vi "Interface _Envio_Recepcion.vi"() -> ()   [LabVIEW 2017]
uses:
  <vilib>/Instr/_visa.llb/VISA Configure Serial Port (Instr).vi
panel:
  out "Acelerómetro Carga 4":waveform(dbl)(graph)
  out "Acelerómetro Eje 2":waveform(dbl)(graph)
  out "Acelerómetro Eje 3":waveform(dbl)(graph)
  out "return count":u32
  in  "Delay":u32
  out "Acelerómetro Motor 1":waveform(dbl)(graph)
  in  "Resetear Gráficos":bool
  out "Datos Crudos":string
  in  "Paro de emergencia":bool
  out "Status":bool
  out "Tasa de muestreo (Hz)":dbl(knob) scale=0.0..1.0
  in  "Puerto COM":refnum<visa-resource-name>
  out "String":string
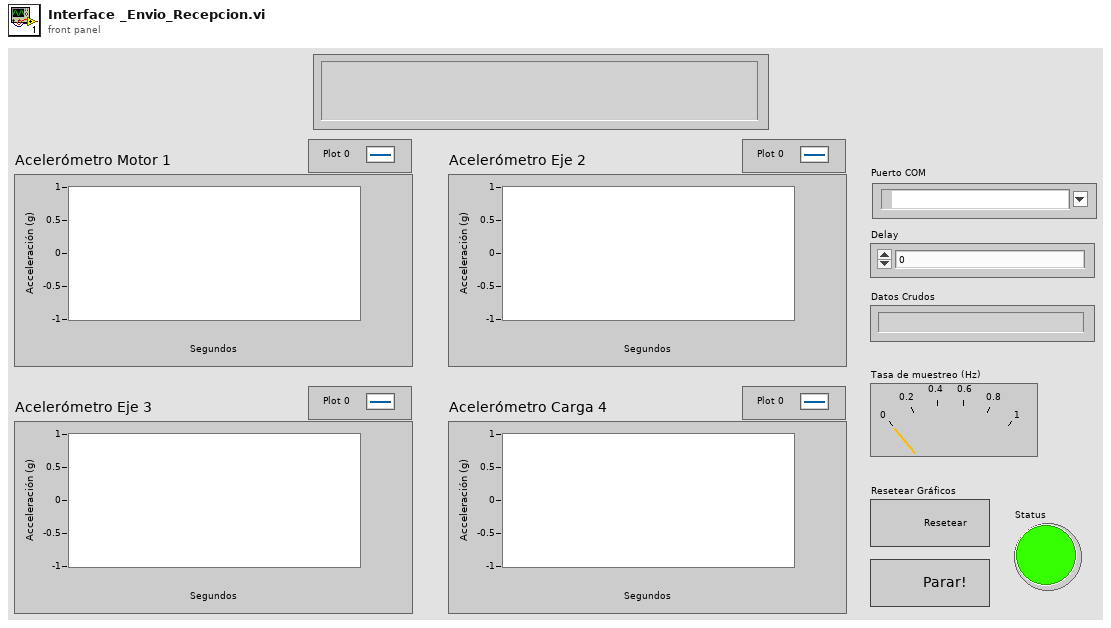
[diagram p1: front panel]
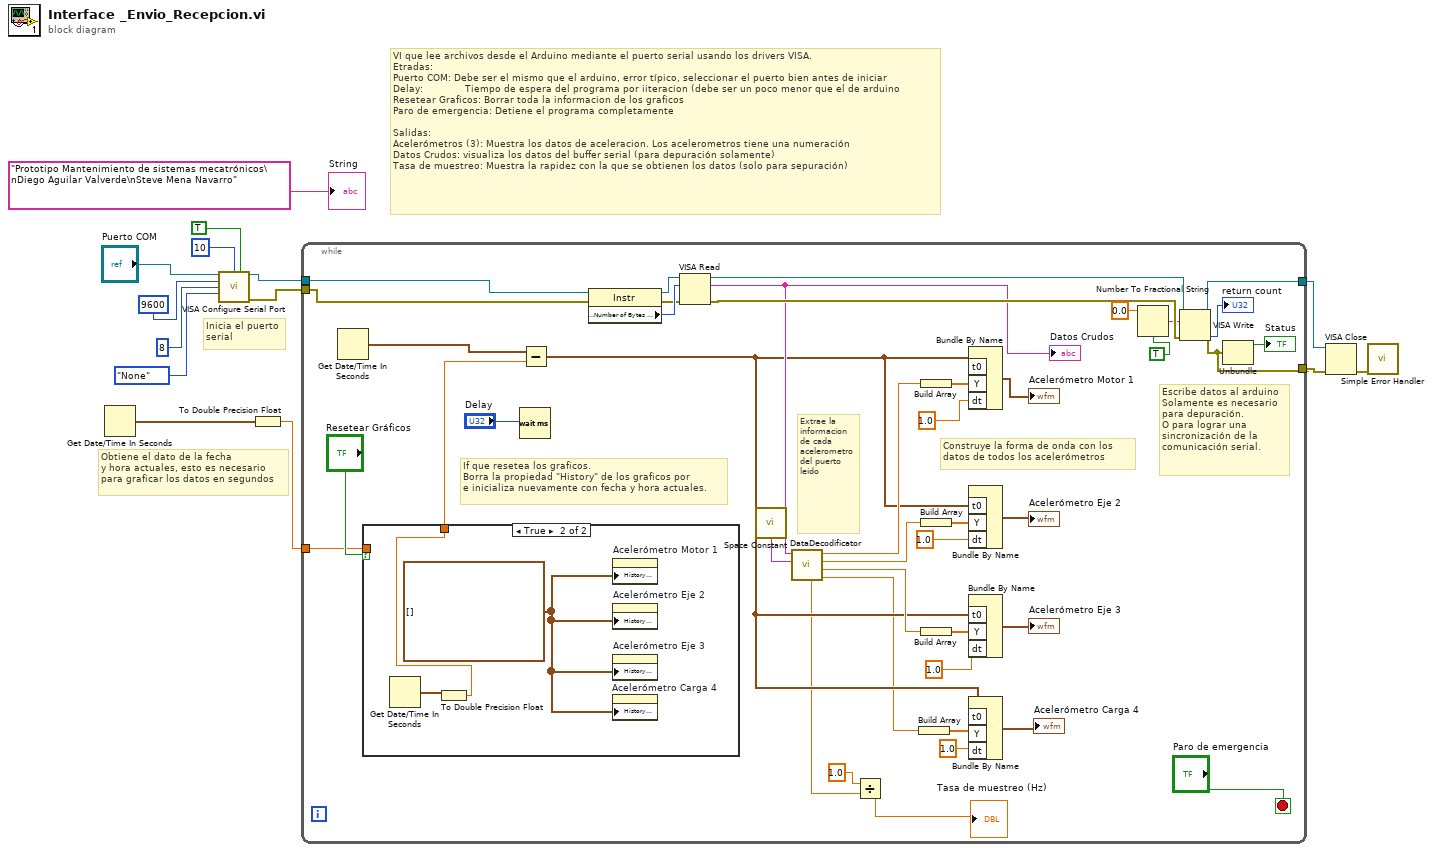
[diagram p0: block diagram]
diagram:
  # "Obtiene el dato de la fecha \ny hora actuales, esto es necesario\npara graficar los datos en segundos"
  # "Inicia el puerto\nserial"
  # "VI que lee archivos desde el Arduino mediante el puerto serial usando los drivers VISA.\nEtradas:\nPuerto COM: Debe ser el mismo que el arduino, error típico, seleccionar el puerto bien antes de iniciar\nDelay:              Tiempo de espera del programa por iiteracion (debe ser un poco menor que el de arduino\nResetear Graficos: Borrar toda la informacion de los graficos\nParo de emergencia: Detiene el programa completamente\n\nSalidas: \nAcelerómetros (3): Muestra los datos de aceleracion. Los acelerometros tiene una numeración\nDatos Crudos: visualiza los datos del buffer serial (para depuración solamente)\nTasa de muestreo: Muestra la rapidez con la que se obtienen los datos (solo para sepuración)"
  n1 = Get Date/Time In Seconds() -> (seconds since 1Jan1904=w1:timestamp)
  n2 = call-poly "VISA Configure Serial Port"("VISA resource name"="Puerto COM", "termination char\n(0xA = '\\n' = LF)"=u8 10 ("termination char\n(0xA = '\\n' = LF)"), "Enable Termination\nChar (T)"=TRUE ("Enable Termination\nChar (T)"), "baud rate (9600)"=u32 9600, "data bits (8)"=u16 8, "parity (0:none)"=enum16{"None", "Odd", "Even", "Mark", "Space"}."None") -> ("VISA resource name out"=w8:refnum<visa-resource-name>, "error out"=w7:errorcluster)  [unwired: 8 in]
  n3 = To Double Precision Float(number=w1) -> (double precision float=w2:dbl)
  n4 = while {
    tunnel: w8 -> [w56]
    tunnel: w7 -> [w55]
    tunnel: [w37] -> w6
    tunnel: [w35] -> w5
    tunnel: w2 -> [w40]
    stop <- "Paro de emergencia" stop-if-true
    # "Escribe datos al arduino\nSolamente es necesario \npara depuración. \nO para lograr una \nsincronización de la \ncomunicación serial."
    # "Extrae la informacion de cada acelerometro del puerto leído"
    # "Construye la forma de onda con los \ndatos de todos los acelerómetros"
    # "If que resetea los graficos.\nBorra la propiedad \"History\" de los graficos por\ne inicializa nuevamente con fecha y hora actuales."
    n5 = Get Date/Time In Seconds() -> (seconds since 1Jan1904=w45:timestamp)
    n6 = case shown="True" "Resetear Gráficos" {
      tunnel: w40 -> [w57 _]
      tunnel: [w57 w59] -> w39
      frame False {
      }
      frame True {
        w58 = waveform(dbl)[] [] ("History Data")
        n7 = Get Date/Time In Seconds() -> (seconds since 1Jan1904=w60:timestamp)
        n8 = To Double Precision Float(number=w60) -> (double precision float=w59:dbl)
        n9 = property on="Acelerómetro Motor 1" class="WFChart (strict)"("History Data"=w58) -> ()  [unwired: 2 in, 2 out]
        n10 = property on="Acelerómetro Eje 2" class="WFChart (strict)"("History Data"=w58) -> ()  [unwired: 2 in, 2 out]
        n11 = property on="Acelerómetro Eje 3" class="WFChart (strict)"("History Data"=w58) -> ()  [unwired: 2 in, 2 out]
        n12 = property on="Acelerómetro Carga 4" class="WFChart (strict)"("History Data"=w58) -> ()  [unwired: 2 in, 2 out]
      }
    }
    n13 = Wait (ms)(milliseconds to wait="Delay") -> ()  [unwired: 1 out]
    n14 = Subtract(x=w45, y=w39) -> (x-y=w22:timestamp)
    n15 = property class="Instr"(reference=w56, error in=w55) -> (reference out=w54:refnum<visa-resource-name>, error out=w52:errorcluster, "Serial Settings:Number of Bytes at Serial Port"=w53:u32)
    n16 = VISA Read(VISA resource name=w54, byte count=w53, error in (no error)=w52) -> (VISA resource name out=w38:refnum<visa-resource-name>, read buffer=w32:string, error out=w36:errorcluster)  [unwired: 1 out]
    "Datos Crudos" <- w32
    n17 = call <vilib>:"Space Constant.vi"() -> ("String"=w48:string)
    n18 = call "DataDecodificator.vi"("Separation Character"=w48, "Read Buffer"=w32) -> ("Load Accel 4"=w19:dbl, "Bearing Accel 3"=w24:dbl, "Bearing Accel 2"=w28:dbl, "Motor Accel 1"=w29:dbl, "Data Rate"=w21:dbl)  [unwired: 5 in]
    n19 = Divide(x=1.0, y=w21) -> (x/y=→"Tasa de muestreo (Hz)":dbl)
    n20 = Build Array(w19) -> (w20:dbl[])
    n21 = Build Array(w29) -> (w47:dbl[])
    n22 = Build Array(w28) -> (w43:dbl[])
    n23 = Build Array(w24) -> (w26:dbl[])
    n24 = Bundle By Name("t0"=w22, "Y"=w47, "dt"=1.0) -> (→"Acelerómetro Motor 1":waveform(dbl))  [unwired: 1 in]
    n25 = Bundle By Name("t0"=w22, "Y"=w43, "dt"=1.0) -> (→"Acelerómetro Eje 2":waveform(dbl))  [unwired: 1 in]
    n26 = Bundle By Name("t0"=w22, "Y"=w26, "dt"=1.0) -> (→"Acelerómetro Eje 3":waveform(dbl))  [unwired: 1 in]
    n27 = Bundle By Name("t0"=w22, "Y"=w20, "dt"=1.0) -> (→"Acelerómetro Carga 4":waveform(dbl))  [unwired: 1 in]
    n28 = Number To Fractional String(use system decimal point (T)=TRUE, number=0.0) -> (F-format string=w33:string)  [unwired: 2 in]
    n29 = VISA Write(VISA resource name=w38, write buffer=w33, error in (no error)=w36) -> (VISA resource name out=w37:refnum<visa-resource-name>, return count=→"return count":u32, error out=w35:errorcluster)
    n30 = Unbundle(w35) -> ("status"=→"Status":bool)  [unwired: 2 out]
  }
  n31 = VISA Close(VISA resource name=w6, error in (no error)=w5) -> (error out=w4:errorcluster)
  n32 = call <vilib>:"Simple Error Handler.vi"("error in (no error)"=w4) -> ()  [unwired: 4 in, 5 out]
  "String" <- "Prototipo Mantenimiento de sistemas mecatrónicos\nDiego Aguilar Valverde\nSteve Mena Navarro"
